vi "view programs.vi"(8 "error in (no error)":errorcluster, 9 "Program":u16(ring) items=["Part-1 - Copy", "Part-1", "z"], 10 "Program List":string[](array[string]), 11 "Programs in":refnum<class "Programs.lvclass">) -> (0 "error out":errorcluster, 2 "Data out":T1, 3 "Programs out":refnum<class "Programs.lvclass">)   [LabVIEW 2025, in "Programs.lvclass"]
uses:
  Programs.lvclass
  Controls/Sequencer/sequence array.ctl
  Controls/Sequencer/step cluster.ctl
  Controls/Sequencer/action enum.ctl
  96def6f4-9641-4b3f-bc78-533ef0ba0b65.vi
  <vilib>/JDP Science/JSONtext/JSON text to Variant.vi
  <vilib>/JDP Science/JSONtext/LVClass Serializer/JSONtext LVClass Serializer.lvclass
  Programs.lvclass/Programs.ctl
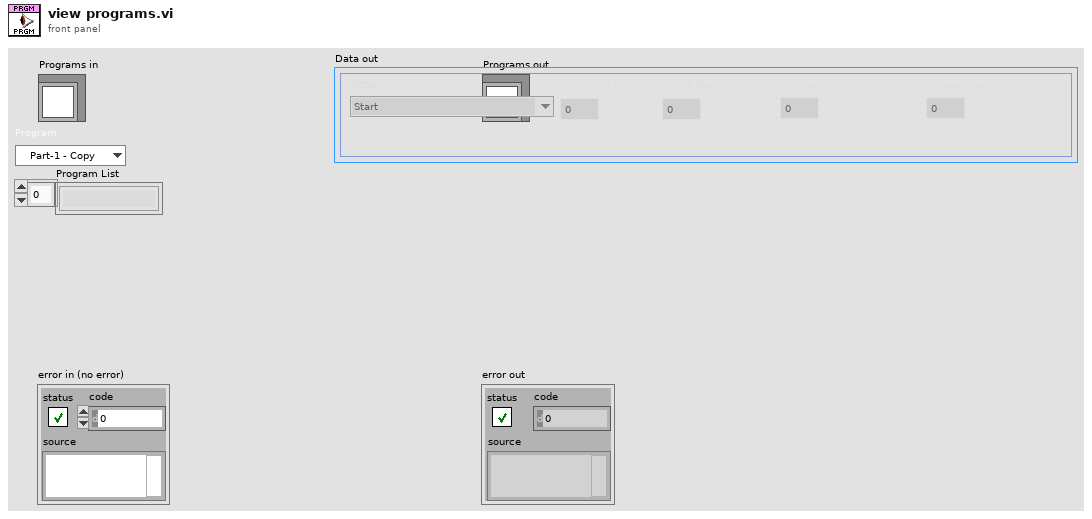
[diagram p1: front panel]
types:
  T1 = typedef "sequence array.ctl" = T2[]
  T2 = typedef "step cluster.ctl" = cluster{"Action":T3, "Angle Min [°]":dbl, "Angle Max [°]":dbl, "Torque Min [oz-in]":dbl, "Torque Max [oz-in]":dbl}
  T3 = typedef "action enum.ctl" = enum16{"Start", "Angle", "Return to Home", "End"}
  T4 = enum16{"open", "replace", "create", "open or create", "replace or create", "replace or create with confirmation"}
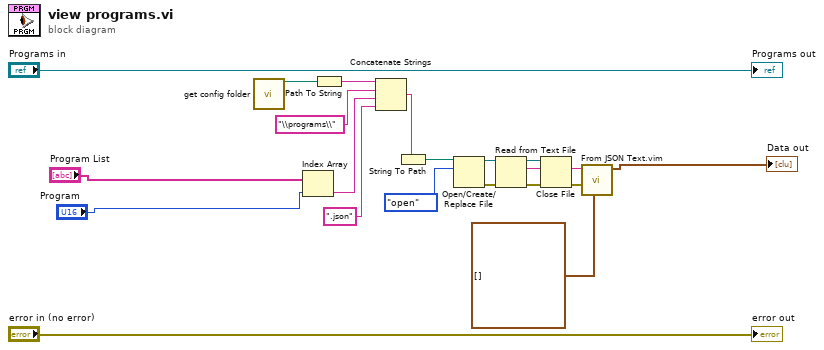
[diagram p0: block diagram]
diagram:
  n1 = call "get config folder.vi"() -> ("Config folder path"=w7:path)  [unwired: 11 in]
  n2 = Index Array(array="Program List", index="Program") -> (element=w6:string)
  n3 = Path To String(path=w7) -> (string=w8:string)
  n4 = Concatenate Strings(w8, "\\programs\\" ("string"), w6, ".json" ("string")) -> (w2:string)
  n5 = String To Path(string=w2) -> (path=w3:path)
  n6 = Open/Create/Replace File(file path (use dialog)=w3, operation (0:open)=T4."open") -> (refnum out=w14:refnum<file>, error out=w13:errorcluster)  [unwired: 4 in, 1 out]
  n7 = Read from Text File(file (use dialog)=w14, error in=w13) -> (refnum out=w11:refnum<file>, text=w15:string, error out=w12:errorcluster)  [unwired: 2 in, 1 out]
  n8 = Close File(refnum=w11, error in=w12) -> (error out=w10:errorcluster)  [unwired: 1 out]
  n9 = call "From JSON Text.vim"("Data Type and Default Value"=T1 [] ("array w/ subset deleted"), "error in (no error)"=w10, "JSON"=w15) -> ("Data out"=→"Data out":T1)  [unwired: 7 in, 1 out]
  "error out" <- "error in (no error)"
  "Programs out" <- "Programs in"
